vi "Teleop.vi"(10 "Match Info":T1={"Autonomous Elapsed Seconds"=0.0, "TeleOp Elapsed Seconds"=0.0, "Disabled Elapsed Seconds"=0.0, "Visited Autonomous"=FALSE, "Visited TeleOp"=FALSE, "Visited Disabled"=FALSE, "Autonomous Settings"={"Autonomous Style"=enum."Independent", "VI Refnum"=refnum}}, 11 "Call Context":T2) -> ()   [LabVIEW 2012]
doc: "This VI is called for each TeleOp packet received from the DS where the robot is not disabled. It is often used to read from the joysticks and update I/O or to update setpoints for timed control loops. It should complete and return within 20 milliseconds or it may miss DS packets."
uses:
  <vilib>/Rock Robotics/WPI/DriverStation/WPI_DriverStationDerivedRobotMode.ctl
  <vilib>/Rock Robotics/WPI/DriverStation/WPI_DriverStationMatch Info.ctl
  <vilib>/Rock Robotics/WPI/Relay/WPI_RelayValue.ctl
  Robot Global Data.vi
  <vilib>/Rock Robotics/WPI/Joystick/WPI_JoystickGetSetRefNum.vi
panel:
  in  "Deadband":dbl=0.15
  in  "Vertical Constant":dbl=0.5
  in  "Horizontal Constant":dbl=0.9
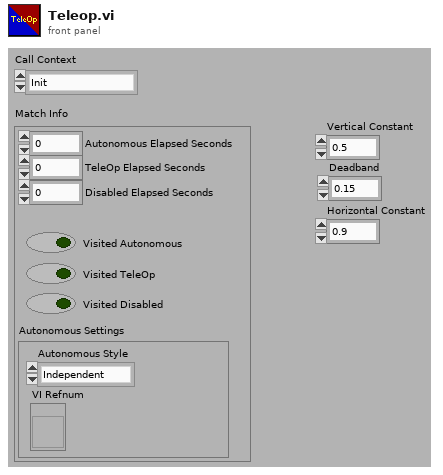
[diagram p1: front panel]
types:
  T1 = typedef "WPI_DriverStationMatch Info.ctl" = cluster{"Autonomous Elapsed Seconds":dbl, "TeleOp Elapsed Seconds":dbl, "Disabled Elapsed Seconds":dbl, "Visited Autonomous":bool, "Visited TeleOp":bool, "Visited Disabled":bool, "Autonomous Settings":cluster{"Autonomous Style":enum16{"Iterative", "Independent"}, "VI Refnum":refnum<vi>}}
  T2 = typedef "WPI_DriverStationDerivedRobotMode.ctl" = enum16{"Init", "Execute", "Stop"}
  T3 = typedef "WPI_RelayValue.ctl" = enum16{"Off", "On", "Forward", "Reverse"}
  T4 = typedef "WPI_JoystickDevRef.ctl" = cluster{"Device":T5}
  T5 = typedef "WPI_JoystickDeviceEnum.ctl" = enum16{"USB 1", "USB 2", "USB 3", "USB 4", "Kinect 1", "Kinect 2"}
  T6 = typedef "WPI_JoystickButtonState.ctl" = cluster{"Button 1":bool, "Button 2":bool, "Button 3":bool, "Button 4":bool, "Button 5":bool, "Button 6":bool, "Button 7":bool, "Button 8":bool, "Button 9":bool, "Button 10":bool, "Button 11":bool, "Button 12":bool}
  T7 = cluster{"axis 1 (x)":dbl, "axis 2 (y)":dbl, "axis 3 (throttle)":dbl, "axis 4":dbl, "axis 5":dbl, "axis 6":dbl}
  T8 = typedef "WPI_RelayDevRef.ctl" = cluster{"DevStatus":errorcluster, "Relay Channel":T9, "Digital Module":T10, "Relay Direction":T11}
  T9 = typedef "FPGA_DIORelayChannel.ctl" = enum8{"Relay 1", "Relay 2", "Relay 3", "Relay 4", "Relay 5", "Relay 6", "Relay 7", "Relay 8", "Invalid"}
  T10 = typedef "FPGA_TypedefDigitalModule.ctl" = enum16{"Digital Module 1", "Digital Module 2"}
  T11 = typedef "WPI_RelayDirection.ctl" = enum16{"Both directions", "Forward only", "Reverse only"}
  T12 = typedef "WPI_MotorControlDeviceRef.ctl" = cluster{"DeviceStatus":errorcluster, "Type":enum16{"PWM", "CAN"}, "PWM":cluster{"Digital Module":T10, "PWM Channel":T13, "DeadBand":T14}, "CAN":cluster{"Device Number":u8, "Control Mode":T15, "Semaphore":T16, "Max Vout":dbl}, "Invert":bool, "TransformRef":T17, "InvTransformRef":T17}
  T13 = typedef "FPGA_DIOPWMChannel.ctl" = enum8{"PWM 1", "PWM 2", "PWM 3", "PWM 4", "PWM 5", "PWM 6", "PWM 7", "PWM 8", "PWM 9", "PWM 10", "Invalid"}
  T14 = typedef "WPI_PWMDeadband.ctl" = cluster{"Name":string, "maxPositivePwm":i32, "minPositivePwm":i32, "centerPwm":i32, "maxNegativePwm":i32, "minNegativePwm":i32, "angularRange":u16}
  T15 = typedef "WPI_CANJaguar_ControlMode.ctl" = enum8{"Percent VBus", "Current", "Speed", "Position", "Voltage"}
  T16 = typedef "Semaphore RefNum" = refnum<k1>
  T17 = typedef "WPI_PWMTransform_ConPane.ctl" = refnum<vi>
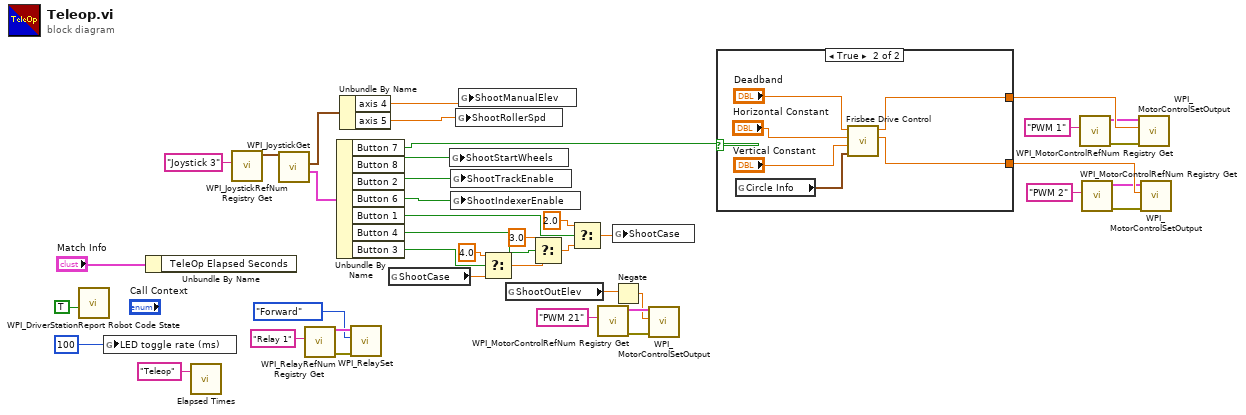
[diagram p0: block diagram]
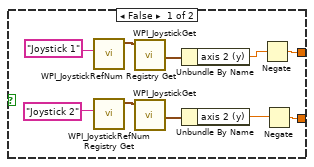
[diagram p2: hidden frame]
diagram:
  n1 = call <vilib>:"WPI_DriverStationReport Robot Code State.vi"("TeleOp"=TRUE ("Autonomous")) -> ()  [unwired: 10 in, 1 out]
  n2 = global write "Robot Global Data.vi" "LED toggle rate (ms)"(u32 100 ("LED ms toggle rate")) -> ()
  n3 = Unbundle By Name("Match Info") -> ()  [unwired: 1 out]
  n4 = call "Elapsed Times.vi"("Call Name"="Teleop") -> ()  [unwired: 2 in, 1 out]
  n5 = call <vilib>:"WPI_JoystickRefNum Registry Get.vi"("refnum name"="Joystick 3") -> ("JoystickDevRef"=w34:T4)  [unwired: 9 in, 1 out]
  n6 = call <vilib>:"WPI_JoystickGet.vi"("JoystickDevRef"=w34) -> ("Buttons"=w32:T6, "Axes"=w31:T7)  [unwired: 4 in, 1 out]
  n7 = call <vilib>:"WPI_RelayRefNum Registry Get.vi"("refnum name"="Relay 1") -> ("error out"=w36:errorcluster, "RelayDevRef"=w38:T8)  [unwired: 9 in]
  n8 = Unbundle By Name(w32) -> ("Button 7"=w1:bool, "Button 8"=w28:bool, "Button 2"=w29:bool, "Button 6"=w30:bool, "Button 1"=w25:bool, "Button 4"=w23:bool, "Button 3"=w22:bool)
  n9 = Unbundle By Name(w31) -> ("axis 4"=w27:dbl, "axis 5"=w26:dbl)
  n10 = call <vilib>:"WPI_RelaySet.vi"("error in (no error)"=w36, "RelayValue"=WPI_RelayValue."Forward", "RelayDevRef"=w38) -> ()  [unwired: 7 in, 2 out]
  n11 = global read "Robot Global Data.vi" "ShootCase"() -> (w17:dbl)
  n12 = global write "Robot Global Data.vi" "ShootStartWheels"(w28) -> ()
  n13 = global write "Robot Global Data.vi" "ShootTrackEnable"(w29) -> ()
  n14 = global write "Robot Global Data.vi" "ShootIndexerEnable"(w30) -> ()
  n15 = global write "Robot Global Data.vi" "ShootRollerSpd"(w26) -> ()
  n16 = global write "Robot Global Data.vi" "ShootManualElev"(w27) -> ()
  n17 = Select(t=4.0, s=w22, f=w17) -> (s? t:f=w21:dbl)
  n18 = global read "Robot Global Data.vi" "ShootOutElev"() -> (w12:dbl)
  n19 = Select(t=3.0, s=w23, f=w21) -> (s? t:f=w19:dbl)
  n20 = Select(t=2.0, s=w25, f=w19) -> (s? t:f=w16:dbl)
  n21 = call <vilib>:"WPI_MotorControlRefNum Registry Get.vi"("refnum name"="PWM 21") -> ("error out"=w15:errorcluster, "MotorControlDevRef"=w14:T12)  [unwired: 9 in]
  n22 = global write "Robot Global Data.vi" "ShootCase"(w16) -> ()
  n23 = Negate(x=w12) -> (-x=w11:dbl)
  n24 = call <vilib>:"WPI_MotorControlSetOutput.vi"("error in (no error)"=w15, "Output"=w11, "MotorControlDevRef"=w14) -> ()  [unwired: 6 in, 3 out]
  n25 = case shown="True" w1 {
    tunnel: [w43 w56] -> w7
    tunnel: [w42 w55] -> w6
    frame False {
      n26 = call <vilib>:"WPI_JoystickRefNum Registry Get.vi"("refnum name"="Joystick 1") -> ("JoystickDevRef"=w50:T4)  [unwired: 1 in, 9 out]
      n27 = call <vilib>:"WPI_JoystickRefNum Registry Get.vi"("refnum name"="Joystick 2") -> ("JoystickDevRef"=w47:T4)  [unwired: 1 in, 9 out]
      n28 = call <vilib>:"WPI_JoystickGet.vi"("JoystickDevRef"=w50) -> ("Axes"=w49:T7)  [unwired: 1 in, 5 out]
      n29 = call <vilib>:"WPI_JoystickGet.vi"("JoystickDevRef"=w47) -> ("Axes"=w48:T7)  [unwired: 1 in, 5 out]
      n30 = Unbundle By Name(w49) -> ("axis 2 (y)"=w44:dbl)
      n31 = Unbundle By Name(w48) -> ("axis 2 (y)"=w45:dbl)
      n32 = Negate(x=w44) -> (-x=w42:dbl)
      n33 = Negate(x=w45) -> (-x=w43:dbl)
    }
    frame True {
      n34 = global read "Robot Global Data.vi" "Circle Info"() -> (w52:cluster{dbl, dbl})
      n35 = call "Frisbee Drive Control.vi"("Circle Info"=w52, "Vertical Constant"="Vertical Constant", "Horizontal Constant"="Horizontal Constant", "Deadband"="Deadband") -> ("Right Drive"=w56:dbl, "Left Drive"=w55:dbl)  [unwired: 6 in]
    }
  }
  n36 = call <vilib>:"WPI_MotorControlRefNum Registry Get.vi"("refnum name"="PWM 1") -> ("error out"=w4:errorcluster, "MotorControlDevRef"=w5:T12)  [unwired: 9 in]
  n37 = call <vilib>:"WPI_MotorControlRefNum Registry Get.vi"("refnum name"="PWM 2") -> ("error out"=w8:errorcluster, "MotorControlDevRef"=w3:T12)  [unwired: 9 in]
  n38 = call <vilib>:"WPI_MotorControlSetOutput.vi"("error in (no error)"=w4, "Output"=w6, "MotorControlDevRef"=w5) -> ()  [unwired: 6 in, 3 out]
  n39 = call <vilib>:"WPI_MotorControlSetOutput.vi"("error in (no error)"=w8, "Output"=w7, "MotorControlDevRef"=w3) -> ()  [unwired: 6 in, 3 out]
